vi "display error and abort.vi"(8 "error in":errorcluster, 9 "Pass":bool, 10 "signal":string) -> (0 "error out":errorcluster)   [LabVIEW 2020]
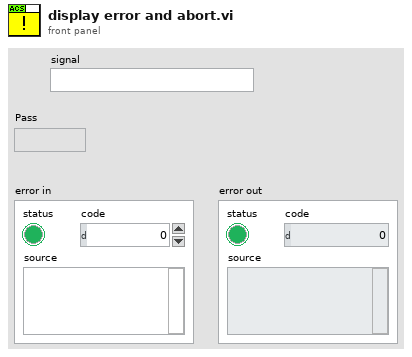
[diagram p1: front panel]
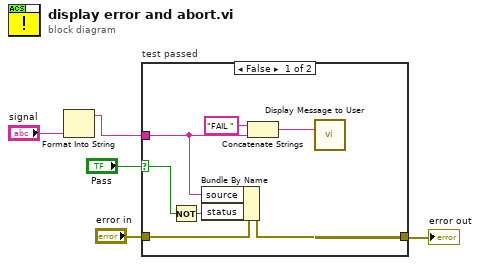
[diagram p0: block diagram]
diagram:
  n1 = Format Into String("signal") -> (resulting string=w1:string)  [unwired: 3 in, 1 out]
  n2 = case "test passed" shown="False" "Pass" {
    selector: "Pass" -> [w9 _]
    tunnel: "error in" -> [w12 w13]
    tunnel: [w11 w13] -> w3
    tunnel: w1 -> [w6 _]
    frame False {
      n3 = Not(x=w9) -> (.not. x?=w10:bool)
      n4 = Bundle By Name(cluster=w12, "source"=w6, "status"=w10) -> (w11:errorcluster)
      n5 = Concatenate Strings("FAIL " ("string"), w6) -> (w7:string)
      n6 = call "Display Message to User"("Message"=w7) -> ()  [unwired: 9 in, 2 out]
    }
    frame True {
    }
  }
  "error out" <- w3
